vi "LS336FrontPanel.vi"() -> ()   [LabVIEW 2020]
uses:
  LS336 FrontPanel/LS336SetTemp.ctl
  LS336 FrontPanel/LS336SetRate.ctl
panel:
  in  "Output 2":u16(ring) items=["A", "B", "C", "D", "None"]
  in  "Output 1":u16(ring) items=["A", "B", "C", "D", "None"]
  in  "VISA resource name":refnum<visa-resource-name>
  in  "stop":bool
  in  "D Rate":T1 caption="K/min" min=0.0 max=50.0 format="%_5g"
  in  "D setp":T2 caption="K" min=0.0 max=350.0 format="%_5g"
  out "D temp":dbl caption="K" format="%.4g"
  in  "C Rate":T1 caption="K/min" min=0.0 max=50.0 format="%_5g"
  in  "C setp":T2 caption="K" min=0.0 max=350.0 format="%_5g"
  out "C temp":dbl caption="K" format="%.4g"
  in  "B Rate":T1 caption="K/min" min=0.0 max=50.0 format="%_5g"
  in  "B setp":T2 caption="K" min=0.0 max=350.0 format="%_5g"
  out "B temp":dbl caption="K" format="%.4g"
  in  "A Rate":T1 caption="K/min" min=0.0 max=50.0 format="%_5g"
  in  "A setp":T2 caption="K" min=0.0 max=350.0 format="%_5g"
  out "A temp":dbl caption="K" format="%.4g"
  # "A"
  # "B"
  # "SETPOINT"
  # "SETPOINT"
  # "RATE"
  # "RATE"
  # "C"
  # "D"
  # "SETPOINT"
  # "SETPOINT"
  # "RATE"
  # "RATE"
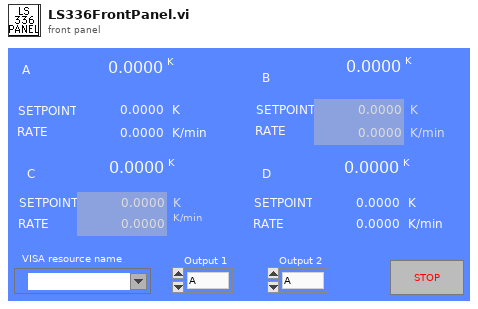
[diagram p1: front panel]
types:
  T1 = typedef "LS336SetRate.ctl" = dbl
  T2 = typedef "LS336SetTemp.ctl" = dbl
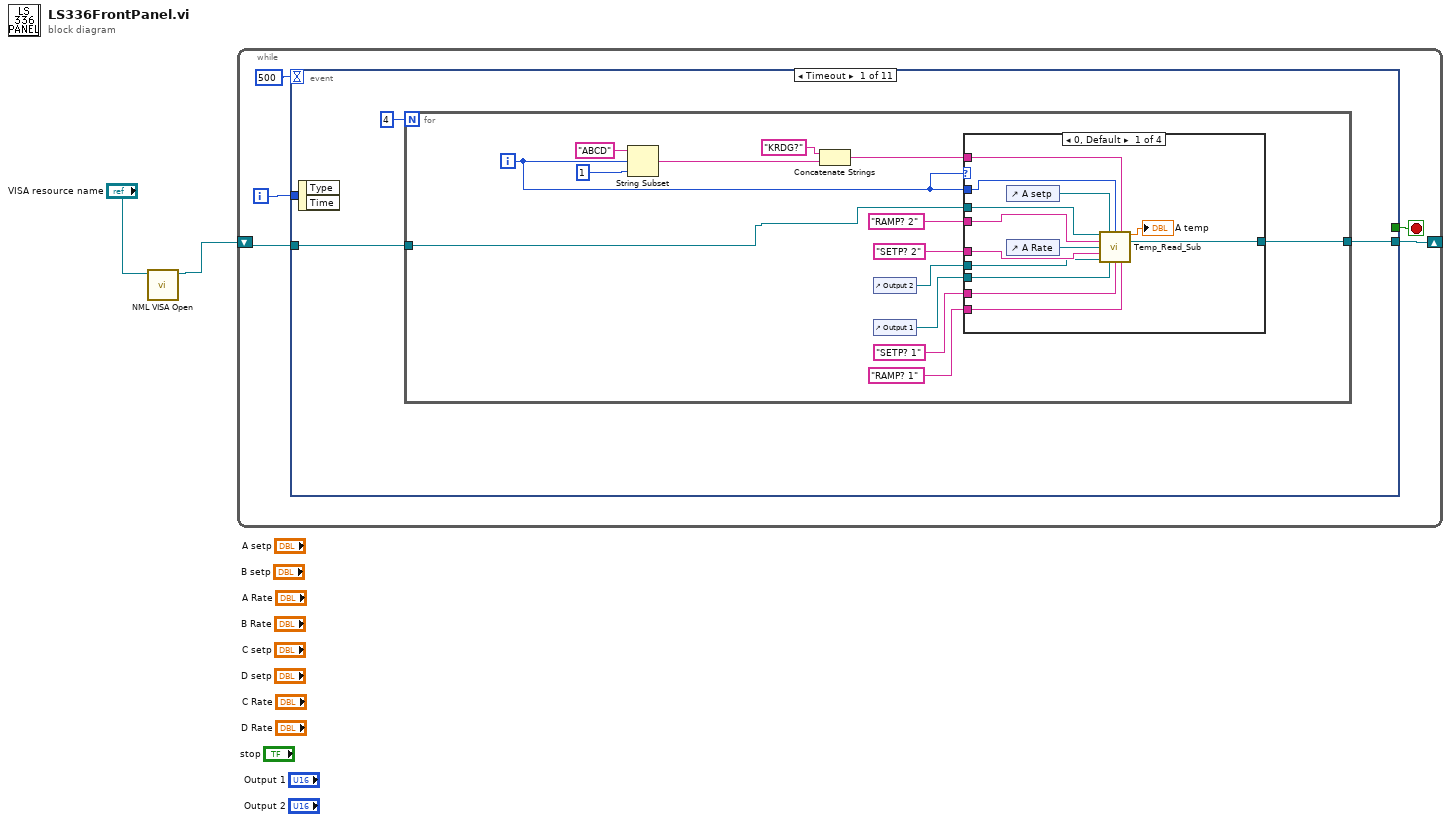
[diagram p0: block diagram]
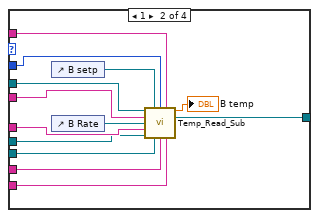
[diagram p2: hidden frame]
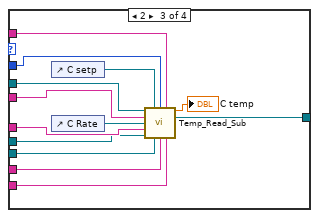
[diagram p3: hidden frame]
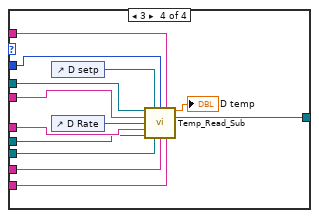
[diagram p4: hidden frame]
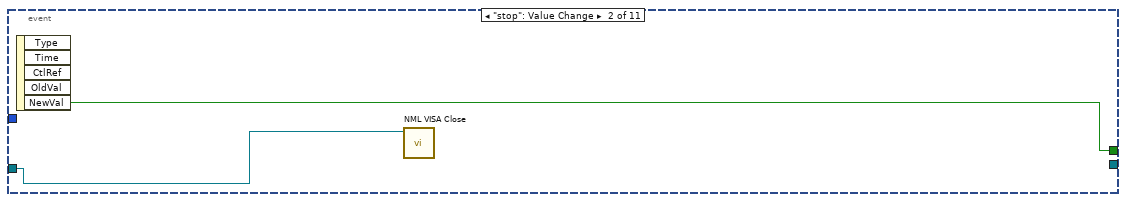
[diagram p5: hidden frame]
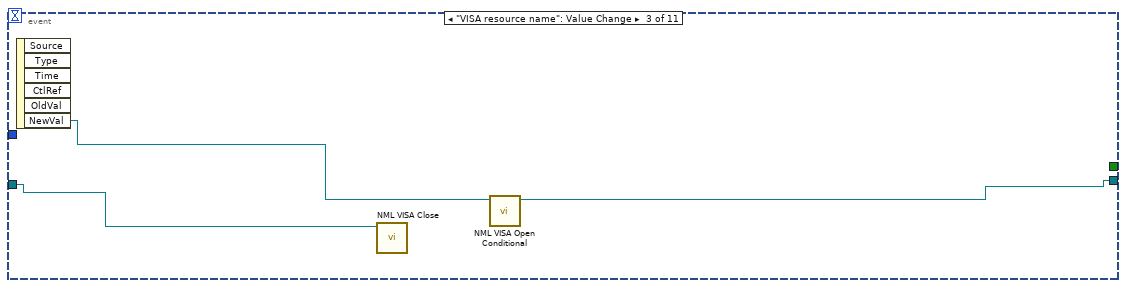
[diagram p6: hidden frame]
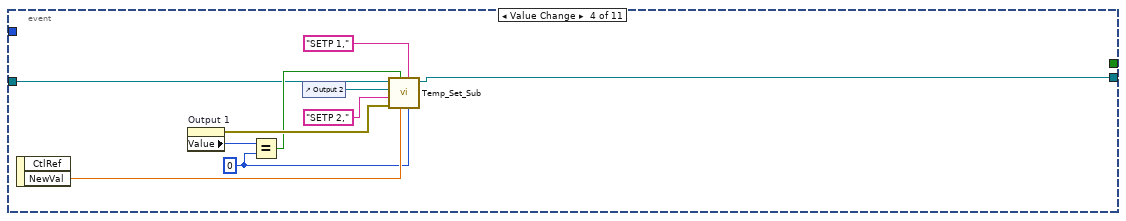
[diagram p7: hidden frame]
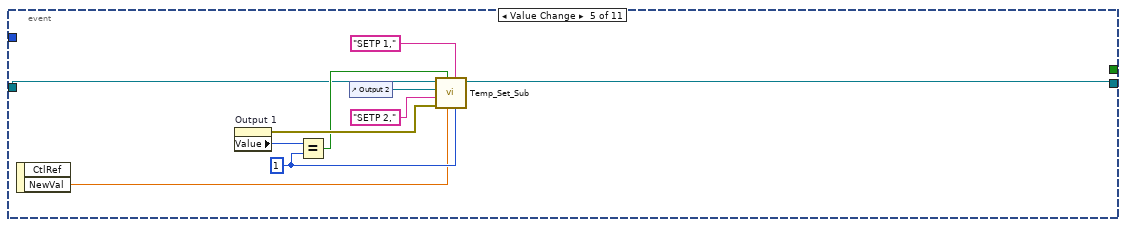
[diagram p8: hidden frame]
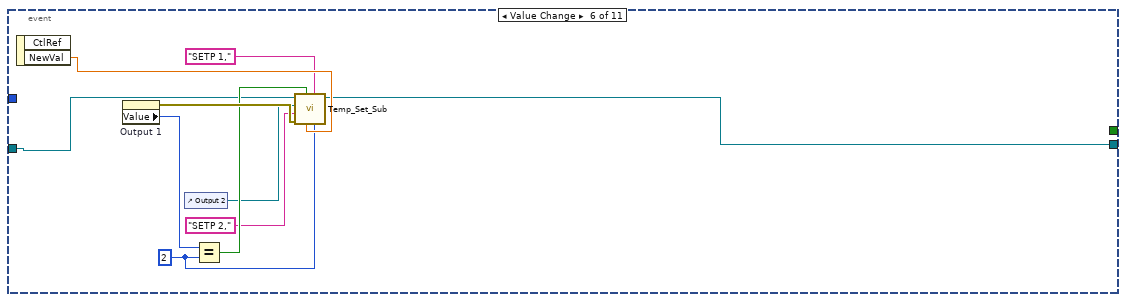
[diagram p9: hidden frame]
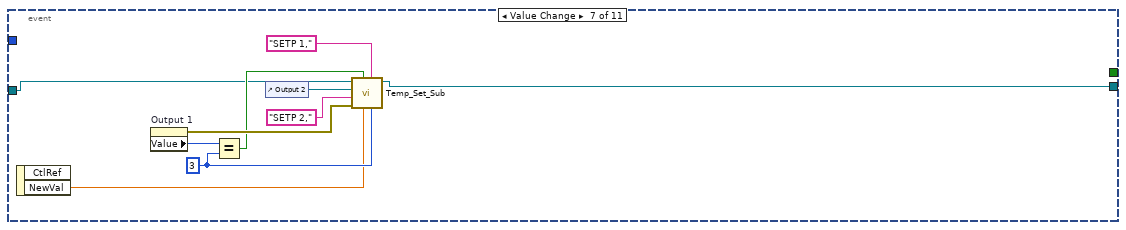
[diagram p10: hidden frame]
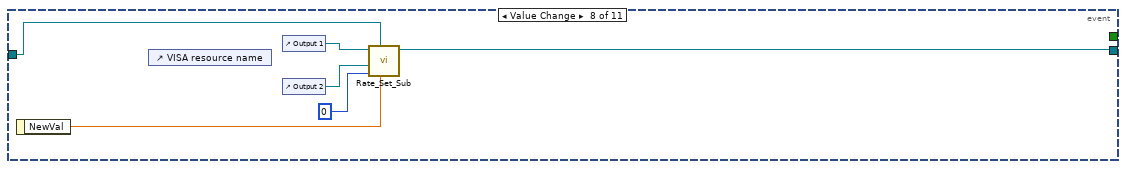
[diagram p11: hidden frame]
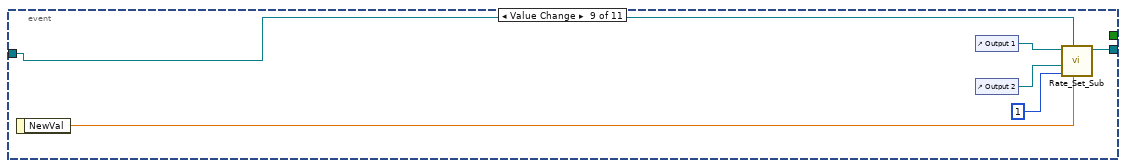
[diagram p12: hidden frame]
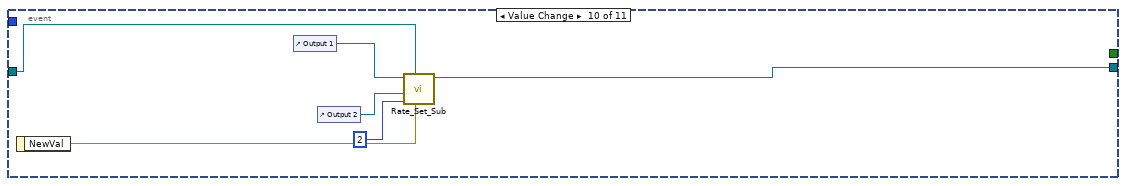
[diagram p13: hidden frame]
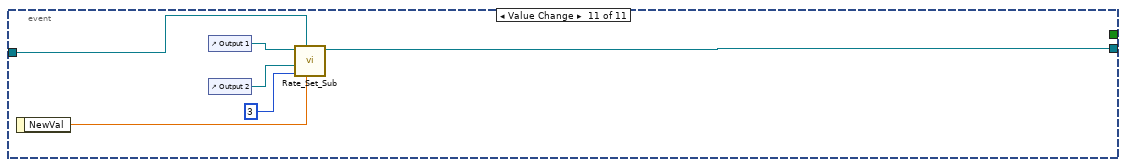
[diagram p14: hidden frame]
diagram:
  n1 = call "NML VISA Open.vi"("VISA resource name"="VISA resource name") -> ("VISA resource name out"=w1:refnum<visa-resource-name>)  [unwired: 9 in, 1 out]
  n2 = while {
    shift-right: [w4] -> _
    shift-left: w1 -> [w3]
    i -> [w7]
    stop <- w6 stop-if-true
    n3 = event shown="[0] Timeout" {
      selector: _ -> [_ _ _ _ _ _ _ _ _ _ _]
      dyn-events: _ -> [_ _ _ _ _ _ _ _ _ _ _]
      timeout: 500 -> [_ _ _ _ _ _ _ _ _ _ _]
      tunnel: w7 -> [_ _ _ _ _ _ _ _ _ _ _]
      tunnel: [_ w78 _ _ _ _ _ _ _ _ _] -> w6
      tunnel: [w9 _ w79 w83 w93 w103 w113 w123 w129 w135 w141] -> w4
      tunnel: w3 -> [w8 w77 w81 w82 w92 w102 w112 w122 w128 w134 w140]
      event Timeout {
        n4 = event-data() -> ()  [unwired: 1 in, 2 out]
        n5 = for {
          N: 4 -> [_]
          tunnel: [w12] -> w9
          tunnel: w8 -> [w11]
          i -> [w23]
          n6 = String Subset(string="ABCD", offset (0)=w23, length (rest)=1 ("length (rest)")) -> (substring=w20:string)
          n7 = Concatenate Strings("KRDG?" ("string"), w20) -> (w21:string)
          n8 = control-ref of="Output 2"() -> (w14:refnum<vi>)
          n9 = control-ref of="Output 1"() -> (w13:refnum<vi>)
          n10 = case shown="0, Default" w23 {
            tunnel: w11 -> [w37 w50 w63 w76]
            tunnel: w23 -> [w36 w49 w62 w75]
            tunnel: w21 -> [w35 w48 w61 w74]
            tunnel: "SETP? 1" ("String to Write") -> [w34 w47 w60 w73]
            tunnel: "RAMP? 1" ("String to Write") -> [w33 w46 w59 w72]
            tunnel: "SETP? 2" ("String to Write") -> [w32 w45 w58 w71]
            tunnel: "RAMP? 2" ("String to Write") -> [w31 w44 w57 w70]
            tunnel: w14 -> [w27 w43 w56 w69]
            tunnel: w13 -> [w26 w42 w55 w68]
            tunnel: [w25 w38 w51 w64] -> w12
            frame 0, Default {
              n11 = control-ref of="A setp"() -> (w30:refnum<vi>)
              n12 = control-ref of="A Rate"() -> (w29:refnum<vi>)
              n13 = call "Temp_Read_Sub.vi"("VISA Refnum in"=w37, "Setp"=w30, "Numeric"=w36, "String"=w35, "String to Write"=w31, "Rate"=w29, "String to Write 2"=w32, "Ring Refnum"=w27, "Ring Refnum 2"=w26, "String to Write 4"=w34, "String to Write 3"=w33) -> ("Temp"=→"A temp":dbl, "dup VISA Session"=w25:refnum<visa-resource-name>)  [unwired: 3 in]
            }
            frame 1 {
              n14 = control-ref of="B setp"() -> (w41:refnum<vi>)
              n15 = control-ref of="B Rate"() -> (w40:refnum<vi>)
              n16 = call "Temp_Read_Sub.vi"("VISA Refnum in"=w50, "Setp"=w41, "Numeric"=w49, "String"=w48, "String to Write"=w44, "Rate"=w40, "String to Write 2"=w45, "Ring Refnum"=w43, "Ring Refnum 2"=w42, "String to Write 4"=w47, "String to Write 3"=w46) -> ("Temp"=→"B temp":dbl, "dup VISA Session"=w38:refnum<visa-resource-name>)  [unwired: 3 in]
            }
            frame 2 {
              n17 = control-ref of="C setp"() -> (w54:refnum<vi>)
              n18 = control-ref of="C Rate"() -> (w53:refnum<vi>)
              n19 = call "Temp_Read_Sub.vi"("VISA Refnum in"=w63, "Setp"=w54, "Numeric"=w62, "String"=w61, "String to Write"=w57, "Rate"=w53, "String to Write 2"=w58, "Ring Refnum"=w56, "Ring Refnum 2"=w55, "String to Write 4"=w60, "String to Write 3"=w59) -> ("Temp"=→"C temp":dbl, "dup VISA Session"=w51:refnum<visa-resource-name>)  [unwired: 3 in]
            }
            frame 3 {
              n20 = control-ref of="D setp"() -> (w67:refnum<vi>)
              n21 = control-ref of="D Rate"() -> (w66:refnum<vi>)
              n22 = call "Temp_Read_Sub.vi"("VISA Refnum in"=w76, "Setp"=w67, "Numeric"=w75, "String"=w74, "String to Write"=w70, "Rate"=w66, "String to Write 2"=w71, "Ring Refnum"=w69, "Ring Refnum 2"=w68, "String to Write 4"=w73, "String to Write 3"=w72) -> ("Temp"=→"D temp":dbl, "dup VISA Session"=w64:refnum<visa-resource-name>)  [unwired: 3 in]
            }
          }
        }
      }
      event "stop": Value Change {
        n23 = event-data() -> ("NewVal"=w78:bool)  [unwired: 1 in, 4 out]
        n24 = call "NML VISA Close.vi"("VISA resource name"=w77) -> ()  [unwired: 10 in, 1 out]
      }
      event "VISA resource name": Value Change {
        n25 = event-data() -> ("NewVal"=w80:refnum<visa-resource-name>)  [unwired: 1 in, 5 out]
        n26 = call "NML VISA Close.vi"("VISA resource name"=w81) -> ()  [unwired: 10 in, 1 out]
        n27 = call "NML VISA Open Conditional.vi"("VISA resource name"=w80) -> ("dup VISA Session"=w79:refnum<visa-resource-name>)  [unwired: 8 in, 2 out]
      }
      event Value Change {
        w85 = u16 0 ("y")
        n28 = event-data() -> ("NewVal"=w86:T2)  [unwired: 1 in, 1 out]
        n29 = property on="Output 1" class="Ring (strict)"() -> (error out=w90:errorcluster, "Value"=w91:u16)  [unwired: 2 in, 1 out]
        n30 = Equal?(x=w91, y=w85) -> (x = y?=w84:bool)
        n31 = control-ref of="Output 2"() -> (w87:refnum<vi>)
        n32 = call "Temp_Set_Sub.vi"("Numeric"=w85, "String to Write"="SETP 1,", "NewVal"=w86, "Boolean"=w84, "error in (no error)"=w90, "String to Write 2"="SETP 2," ("String to Write"), "Ring Refnum"=w87, "Value"=w82) -> ("dup VISA Session"=w83:refnum<visa-resource-name>)  [unwired: 3 in]
      }
      event Value Change {
        w97 = u16 1 ("y")
        n33 = event-data() -> ("NewVal"=w95:T2)  [unwired: 1 in, 1 out]
        n34 = property on="Output 1" class="Ring (strict)"() -> (error out=w100:errorcluster, "Value"=w101:u16)  [unwired: 2 in, 1 out]
        n35 = Equal?(x=w101, y=w97) -> (x = y?=w98:bool)
        n36 = control-ref of="Output 2"() -> (w96:refnum<vi>)
        n37 = call "Temp_Set_Sub.vi"("Numeric"=w97, "String to Write"="SETP 1,", "NewVal"=w95, "Boolean"=w98, "error in (no error)"=w100, "String to Write 2"="SETP 2," ("String to Write"), "Ring Refnum"=w96, "Value"=w92) -> ("dup VISA Session"=w93:refnum<visa-resource-name>)  [unwired: 3 in]
      }
      event Value Change {
        w104 = u16 2 ("y")
        n38 = event-data() -> ("NewVal"=w109:T2)  [unwired: 1 in, 1 out]
        n39 = property on="Output 1" class="Ring (strict)"() -> (error out=w110:errorcluster, "Value"=w111:u16)  [unwired: 2 in, 1 out]
        n40 = control-ref of="Output 2"() -> (w106:refnum<vi>)
        n41 = Equal?(x=w111, y=w104) -> (x = y?=w107:bool)
        n42 = call "Temp_Set_Sub.vi"("Numeric"=w104, "String to Write"="SETP 1,", "NewVal"=w109, "Boolean"=w107, "error in (no error)"=w110, "String to Write 2"="SETP 2," ("String to Write"), "Ring Refnum"=w106, "Value"=w102) -> ("dup VISA Session"=w103:refnum<visa-resource-name>)  [unwired: 3 in]
      }
      event Value Change {
        w116 = u16 3 ("y")
        n43 = event-data() -> ("NewVal"=w114:T2)  [unwired: 1 in, 1 out]
        n44 = property on="Output 1" class="Ring (strict)"() -> (error out=w120:errorcluster, "Value"=w121:u16)  [unwired: 2 in, 1 out]
        n45 = Equal?(x=w121, y=w116) -> (x = y?=w117:bool)
        n46 = control-ref of="Output 2"() -> (w115:refnum<vi>)
        n47 = call "Temp_Set_Sub.vi"("Numeric"=w116, "String to Write"="SETP 1,", "NewVal"=w114, "Boolean"=w117, "error in (no error)"=w120, "String to Write 2"="SETP 2," ("String to Write"), "Ring Refnum"=w115, "Value"=w112) -> ("dup VISA Session"=w113:refnum<visa-resource-name>)  [unwired: 3 in]
      }
      event Value Change {
        n48 = event-data() -> ("NewVal"=w127:T1)  [unwired: 1 in]
        n49 = control-ref of="VISA resource name"() -> ()  [unwired: 1 out]
        n50 = control-ref of="Output 1"() -> (w126:refnum<vi>)
        n51 = control-ref of="Output 2"() -> (w125:refnum<vi>)
        n52 = call "Rate_Set_Sub.vi"("NewVal"=w127, "VISA resource name"=w122, "Numeric"=0, "Ring Refnum in"=w125, "Ring in"=w126) -> ("dup VISA Session"=w123:refnum<visa-resource-name>)  [unwired: 6 in]
      }
      event Value Change {
        n53 = event-data() -> ("NewVal"=w133:T1)  [unwired: 1 in]
        n54 = control-ref of="Output 1"() -> (w132:refnum<vi>)
        n55 = control-ref of="Output 2"() -> (w131:refnum<vi>)
        n56 = call "Rate_Set_Sub.vi"("NewVal"=w133, "VISA resource name"=w128, "Numeric"=1, "Ring Refnum in"=w131, "Ring in"=w132) -> ("dup VISA Session"=w129:refnum<visa-resource-name>)  [unwired: 6 in]
      }
      event Value Change {
        n57 = event-data() -> ("NewVal"=w139:T1)  [unwired: 1 in]
        n58 = control-ref of="Output 1"() -> (w138:refnum<vi>)
        n59 = control-ref of="Output 2"() -> (w137:refnum<vi>)
        n60 = call "Rate_Set_Sub.vi"("NewVal"=w139, "VISA resource name"=w134, "Numeric"=2, "Ring Refnum in"=w137, "Ring in"=w138) -> ("dup VISA Session"=w135:refnum<visa-resource-name>)  [unwired: 6 in]
      }
      event Value Change {
        n61 = event-data() -> ("NewVal"=w145:T1)  [unwired: 1 in]
        n62 = control-ref of="Output 1"() -> (w144:refnum<vi>)
        n63 = control-ref of="Output 2"() -> (w143:refnum<vi>)
        n64 = call "Rate_Set_Sub.vi"("NewVal"=w145, "VISA resource name"=w140, "Numeric"=3, "Ring Refnum in"=w143, "Ring in"=w144) -> ("dup VISA Session"=w141:refnum<visa-resource-name>)  [unwired: 6 in]
      }
    }
  }
